vi "Next Step.vi"(8 "error in (no error)":errorcluster, 11 "Magnetic Field.lvclass in":refnum<class "Magnetic Field.lvclass">) -> (0 "error out":errorcluster, 1 "Current Step":u32, 2 "actual position":dbl, 3 "Magnetic Field.lvclass out":refnum<class "Magnetic Field.lvclass">)   [LabVIEW 2017, in "Magnetic Field.lvclass"]
uses:
  Magnetic Field.lvclass
  Instruments/Magnet/Power Supply/Power Supply.lvclass
  C:/LabVIEW-programs-dev/Instruments/Utility Classes/Scannable/Scannable.lvclass
  Scanner/Scanner.lvclass
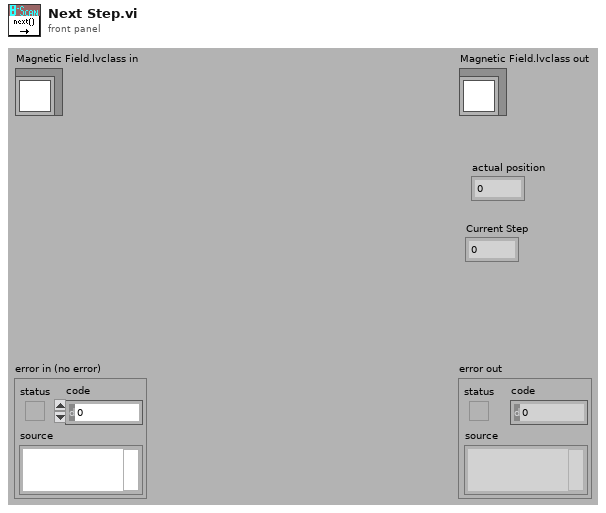
[diagram p1: front panel]
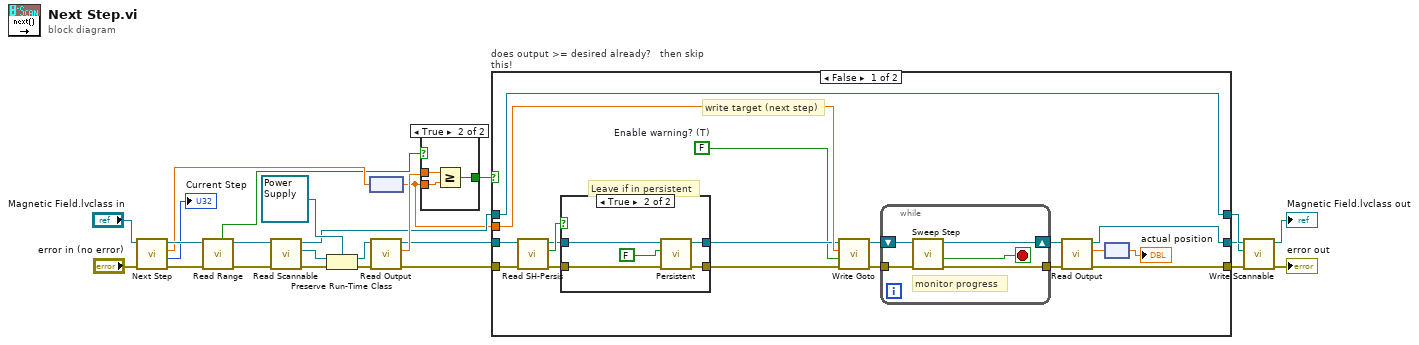
[diagram p0: block diagram]
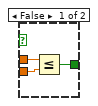
[diagram p2: hidden frame]
diagram:
  n1 = call-parent "Next Step.vi"("error in (no error)"="error in (no error)", "Scanner in"="Magnetic Field.lvclass in") -> ("error out"=w20:errorcluster, "Current Step"=→"Current Step":u32, "Current Position"=w19:dbl, "Scanner out"=w25:refnum<class "Magnetic Field.lvclass">)  [unwired: 6 out]
  n2 = call-dynamic "Read Range.vi"("error in (no error)"=w20, "Scanner.lvclass in"=w25) -> ("error out"=w4:errorcluster, "Scanner.lvclass out"=w13:refnum<class "Magnetic Field.lvclass">, "Scanning Up?"=w17:bool)  [unwired: 7 out]
  n3 = call-dynamic "Read Scannable.vi"("error in (no error)"=w4, "Scanner.lvclass in"=w13) -> ("error out"=w16:errorcluster, "Scannable.lvclass"=w15:refnum<class "Scannable.lvclass">, "Scanner.lvclass out"=w12:refnum<class "Magnetic Field.lvclass">)  [unwired: 7 in]
  n4 = Preserve Run-Time Class(object in=w15, error in=w16, 2:refnum<class "Power Supply.lvclass"> refnum ("Power Supply in")) -> (object out=w6:refnum<class "Power Supply.lvclass">, error out=w1:errorcluster)
  n5 = node(w19) -> (w7:dbl[unit])
  n6 = call-dynamic "Read Output.vi"("error in (no error)"=w1, "Power Supply in"=w6) -> ("error out"=w2:errorcluster, "Field"=w18:dbl[unit], "Power Supply out"=w5:refnum<class "Power Supply.lvclass">)  [unwired: 5 in, 2 out]
  n7 = case shown="True" w17 {
    tunnel: w7 -> [w27 w31]
    tunnel: [w26 w30] -> w21
    tunnel: w18 -> [w28 w29]
    frame False {
      n8 = Less Or Equal?(x=w28, y=w27) -> (x <= y?=w26:bool)
    }
    frame True {
      n9 = Greater Or Equal?(x=w29, y=w31) -> (x >= y?=w30:bool)
    }
  }
  n10 = case "does output >= desired already?   then skip this!" shown="False" w21 {
    tunnel: w7 -> [w49 _]
    tunnel: w12 -> [w44 w64]
    tunnel: [w44 w64] -> w11
    tunnel: w5 -> [w48 w63]
    tunnel: w2 -> [w47 w62]
    tunnel: [w46 w63] -> w10
    tunnel: [w45 w62] -> w9
    frame False {
      w32 = FALSE  # Enable warning? (T)
      # "write target (next step)"
      # "Leave if in persistent"
      n11 = call-dynamic "Read SH-Persis.vi"("error in (no error)"=w47, "Power Supply in"=w48) -> ("error out"=w35:errorcluster, "pers?"=w37:bool, "Power Supply out"=w36:refnum<class "Power Supply.lvclass">)  [unwired: 4 in, 3 out]
      n12 = case shown="True" w37 {
        tunnel: w36 -> [w56 w60]
        tunnel: [w56 w59] -> w40
        tunnel: [w55 w58] -> w39
        tunnel: w35 -> [w55 w57]
        frame False {
        }
        frame True {
          n13 = call-dynamic "Persistent.vi"("error in (no error)"=w57, "Go to persistent mode?"=FALSE, "Power Supply in"=w60) -> ("error out"=w58:errorcluster, "Power Supply out"=w59:refnum<class "Power Supply.lvclass">)  [unwired: 7 in]
        }
      }
      n14 = call-dynamic "Write Goto.vi"("error in (no error)"=w39, "Enable warning? (T)"=w32, "Target"=w49, "Power Supply in"=w40) -> ("error out"=w41:errorcluster, "Power Supply out"=w42:refnum<class "Power Supply.lvclass">)  [unwired: 6 in]
      n15 = while {
        shift-right: [w54] -> w43
        shift-left: w42 -> [w53]
        tunnel: w41 -> [w52]
        tunnel: [w50] -> w38
        stop <- w51 stop-if-true
        # "monitor progress"
        n16 = call-dynamic "Sweep Step.vi"("error in (no error)"=w52, "Power Supply in"=w53) -> ("error out"=w50:errorcluster, "Done?"=w51:bool, "Power Supply out"=w54:refnum<class "Power Supply.lvclass">)  [unwired: 5 in, 2 out]
      }
      n17 = call-dynamic "Read Output.vi"("error in (no error)"=w38, "Power Supply in"=w43) -> ("error out"=w45:errorcluster, "Field"=w34:dbl[unit], "Power Supply out"=w46:refnum<class "Power Supply.lvclass">)  [unwired: 5 in, 2 out]
      n18 = node(w34) -> (→"actual position":dbl)
    }
    frame True {
    }
  }
  n19 = call-dynamic "Write Scannable.vi"("error in (no error)"=w9, "Scannable.lvclass"=w10, "Scanner.lvclass in"=w11) -> ("error out"=→"error out":errorcluster, "Scanner.lvclass out"=→"Magnetic Field.lvclass out":refnum<class "Magnetic Field.lvclass">)  [unwired: 7 in]
